vi "Variant to String Data.vi"(8 "error in (no error)":errorcluster, 11 "Variant":variant) -> (0 "error out":errorcluster, 3 "String Data":string)   [LabVIEW 2014]
uses:
  <vilib>/Utility/error.llb/Error Cluster From Error Code.vi
  <vilib>/ErrorRing/Error Ring.xnode
  <vilib>/Utility/VariantDataType/VariantType.lvlib
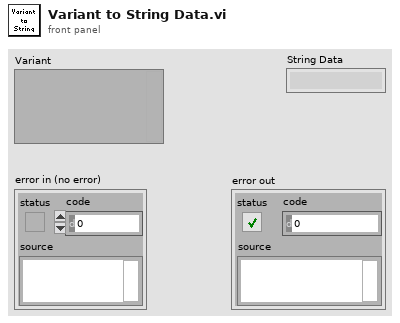
[diagram p1: front panel]
types:
  T1 = typedef "VariantType.lvlib/Type.ctl" = enum8{"Invalid Type", "Void", "I8", "I16", "I32", "I64", "U8", "U16", "U32", "U64", "Single Float", "Double Float", "Extended Float", "Single Complex", "Double Complex", "Extended Complex", "Enum U8", "Enum U16", "Enum U32", "Enum U64", "Single Float With Unit", "Double Float With Unit", "Extended Float With Unit", "Single Complex with Unit", "Double Complex with Unit", "Extended Complex with Unit", "Boolean", "String", "Path", "Picture", "Tag", "Array", "Cluster", "Variant", "LV Variant", "Waveform", "Timestamp", "Digital Waveform", "Digital Data", "ExpressData", "Refnum", "External Data", "VI", "Poly VI", "LabVIEW Class Instance", "Fixed Point"}
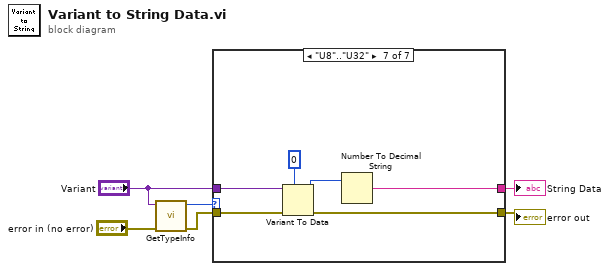
[diagram p0: block diagram]
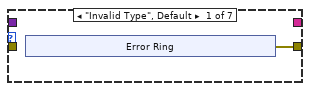
[diagram p2: hidden frame]
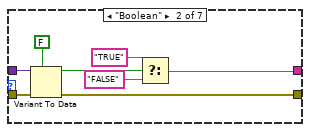
[diagram p3: hidden frame]
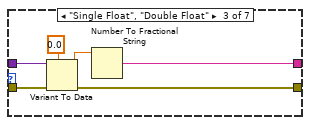
[diagram p4: hidden frame]
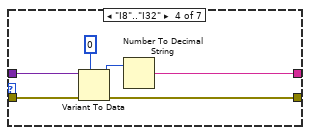
[diagram p5: hidden frame]
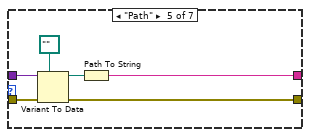
[diagram p6: hidden frame]
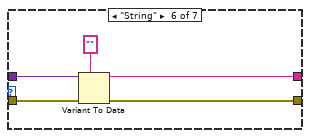
[diagram p7: hidden frame]
diagram:
  n1 = call <vilib>:"GetTypeInfo.vi"("error in (no error)"="error in (no error)", "Variant"="Variant") -> ("error out"=w5:errorcluster, "Type Enum"=w6:T1)  [unwired: 5 in, 3 out]
  n2 = case shown="\"U8\"..\"U32\"" w6 {
    tunnel: "Variant" -> [_ w19 w25 w30 w37 w42 w47]
    tunnel: w5 -> [_ w17 w23 w29 w35 w40 w45]
    tunnel: [w7 w16 w22 w28 w34 w39 w46] -> w1
    tunnel: [_ w12 w20 w26 w32 w38 w44] -> w3
    frame "Invalid Type", Default {
      n3 = xnode "Error Ring"() -> ("error out"=w7:errorcluster)
    }
    frame "Boolean" {
      n4 = Variant To Data(error in=w17, type=FALSE, Variant=w19) -> (data=w15:bool, error out=w16:errorcluster)
      n5 = Select(t="TRUE", s=w15, f="FALSE") -> (s? t:f=w12:string)
    }
    frame "Single Float", "Double Float" {
      n6 = Variant To Data(error in=w23, type=0.0, Variant=w25) -> (data=w21:dbl, error out=w22:errorcluster)
      n7 = Number To Fractional String(number=w21) -> (F-format string=w20:string)  [unwired: 3 in]
    }
    frame "I8".."I32" {
      n8 = Variant To Data(error in=w29, type=0 ("value"), Variant=w30) -> (data=w27:i32, error out=w28:errorcluster)
      n9 = Number To Decimal String(number=w27) -> (decimal integer string=w26:string)  [unwired: 1 in]
    }
    frame "Path" {
      n10 = Variant To Data(error in=w35, type=path "", Variant=w37) -> (data=w33:path, error out=w34:errorcluster)
      n11 = Path To String(path=w33) -> (string=w32:string)
    }
    frame "String" {
      n12 = Variant To Data(error in=w40, type="", Variant=w42) -> (data=w38:string, error out=w39:errorcluster)
    }
    frame "U8".."U32" {
      n13 = Variant To Data(error in=w45, type=u32 0 ("value"), Variant=w47) -> (data=w43:u32, error out=w46:errorcluster)
      n14 = Number To Decimal String(number=w43) -> (decimal integer string=w44:string)  [unwired: 1 in]
    }
  }
  "String Data" <- w3
  "error out" <- w1
